vi "PXI-Get Sync Source.vi"(11 "error in (no error)":errorcluster) -> (4 "Terminal Name with Device Prefix":tag, 15 "error out":errorcluster)   [LabVIEW 2020]
uses:
  <resource>/objmgr/daqmx.rc
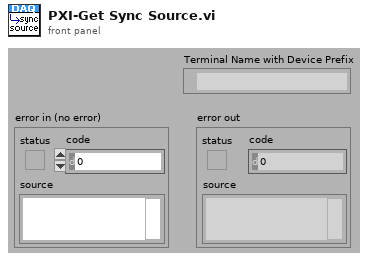
[diagram p1: front panel]
types:
  T1 = cluster{"DAQChan to PhysDev":i32[][], "PhysDev to DAQChan":i32[][]}
  T2 = typedef "Channel Struct.ctl" = cluster{"Channel name":string, "Vmax":dbl, "Vmin":dbl, "Rate":dbl, "Terminal configuration":i32, "Physical Channel":tag, "Regenerate":bool}
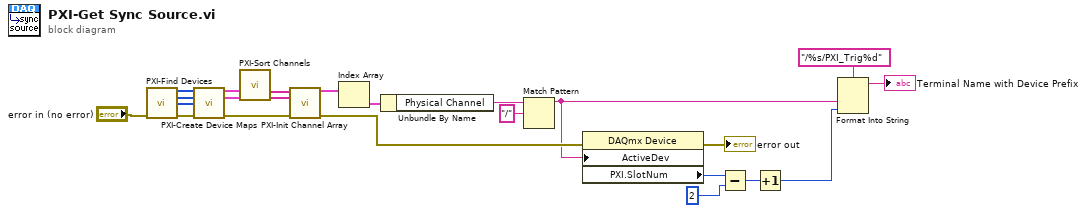
[diagram p0: block diagram]
diagram:
  n1 = call "PXI-Find Devices.vi"("error in (no error)"="error in (no error)") -> ("Num AO"=w21:i32[], "Num AI"=w20:i32[], "Slot Num"=w23:u32[], "error out"=w22:errorcluster)  [unwired: 11 in]
  n2 = call "PXI-Create Device Maps.vi"("Num AO"=w21, "Num AI"=w20, "Slot Num"=w23, "error in (no error)"=w22) -> ("AO Map"=w19:T1, "AI Map"=w18:T1, "error out"=w15:errorcluster)  [unwired: 9 in]
  n3 = call "PXI-Sort Channels.vi"("AO Map"=w19, "AI Map"=w18) -> ("Sorted channel names"=w14:string[], "Sorted physical channels"=w13:tag[])  [unwired: 12 in]
  n4 = call "PXI-Init Channel Array.vi"("Sorted channel names"=w14, "Sorted physical channels"=w13, "error in (no error)"=w15) -> ("Channel Array"=w12:T2[], "error out"=w9:errorcluster)  [unwired: 11 in]
  n5 = Index Array(array=w12) -> (element=w11:T2)  [unwired: 1 in]
  n6 = Unbundle By Name(w11) -> ("Physical Channel"=w10:tag)
  n7 = Match Pattern(string=w10, regular expression="/") -> (before substring=w4:string)  [unwired: 1 in, 3 out]
  n8 = property class="DAQmx Device"(error in=w9, "ActiveDev"=w4) -> (error out=→"error out":errorcluster, "PXI.SlotNum"=w6:u32)  [unwired: 1 in, 1 out]
  n9 = Subtract(x=w6, y=u32 2) -> (x-y=w3:u32)
  n10 = Increment(x=w3) -> (x+1=w1:u32)
  n11 = Format Into String(format string="/%s/PXI_Trig%d", w4, w1) -> (resulting string=→"Terminal Name with Device Prefix":string)  [unwired: 2 in, 1 out]
